vi "Deserialize Connection Info.vi"(7 "Field Delimiter (::)":string="::", 8 "error in (no error)":errorcluster, 11 "Connection Info String":string) -> (0 "error out":errorcluster, 3 "Deserialized Connection Info":T1)   [LabVIEW 2020, in "plugin_flodx_ph_probe.lvlib" / "plugin.lvlib" / "Instrument Manager.lvlib"]
doc: "Deserializes a connection info string. By default, it deserializes a string in the format \"<visa_resource>::<pump_address>\"."
uses:
  Instrument Manager.lvlib
  Connection Info.ctl
panel:
  out "homogenized string":string
  # "Debug"
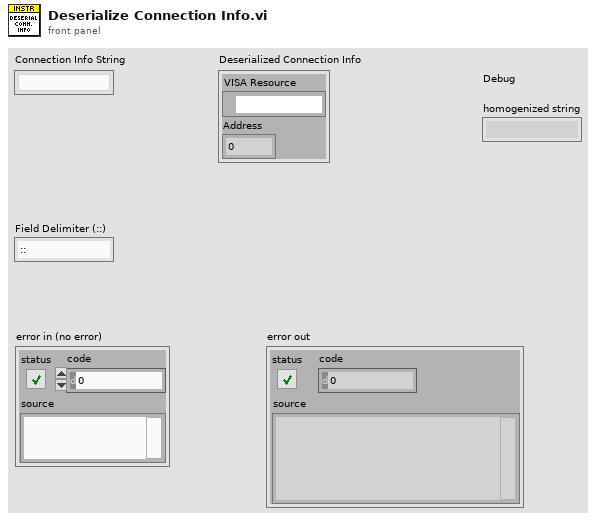
[diagram p1: front panel]
types:
  T1 = typedef "plugin_flodx_ph_probe.lvlib/plugin.lvlib/Instrument Manager.lvlib/Connection Info.ctl" = cluster{"VISA Resource":refnum<visa-resource-name>, "Address":u8}
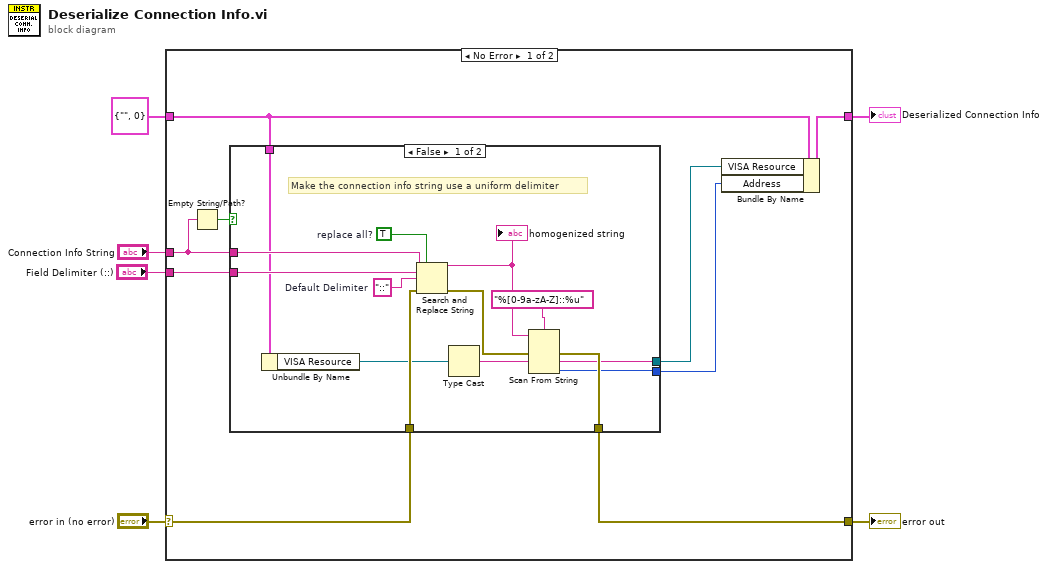
[diagram p0: block diagram]
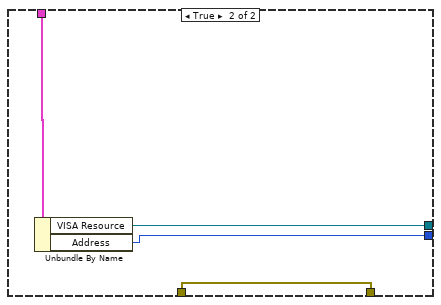
[diagram p2: hidden frame]
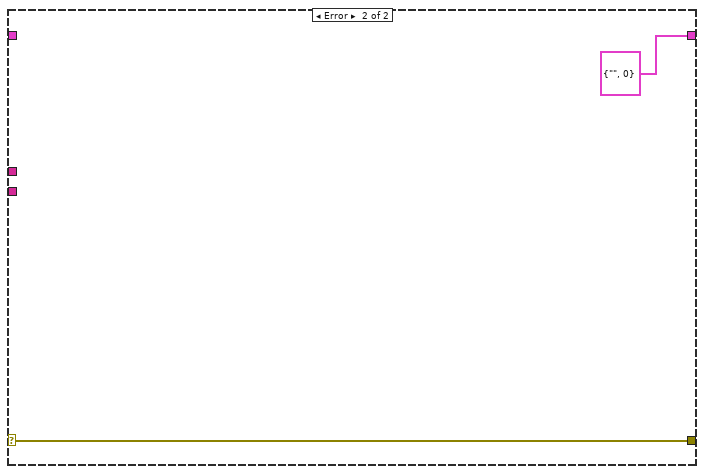
[diagram p3: hidden frame]
diagram:
  n1 = case shown="No Error" "error in (no error)" {
    selector: "error in (no error)" -> [w14 w35]
    tunnel: [w15 w35] -> w5
    tunnel: "Field Delimiter (::)" -> [w13 _]
    tunnel: [w12 T1 {"VISA Resource"="", "Address"=0} ("Deserialized Connection Info")] -> w3
    tunnel: "Connection Info String" -> [w8 _]
    tunnel: T1 {"VISA Resource"="", "Address"=0} ("Deserialized Connection Info") -> [w10 _]
    frame No Error {
      n2 = Empty String/Path?(string/path=w8) -> (empty?=w9:bool)
      n3 = case shown="False" w9 {
        tunnel: [w29 w31] -> w15
        tunnel: w14 -> [w28 w31]
        tunnel: w8 -> [w23 _]
        tunnel: w13 -> [w22 _]
        tunnel: [w19 w32] -> w11
        tunnel: w10 -> [w17 w33]
        tunnel: [w16 w30] -> w7
        frame False {
          w26 = TRUE  # replace all?
          w21 = "::"  # Default Delimiter
          # "Make the connection info string use a uniform delimiter"
          n4 = Unbundle By Name(w17) -> ("VISA Resource"=w25:refnum<visa-resource-name>)
          n5 = Search and Replace String(replace all?=w26, input string=w23, search string=w22, replace string=w21, error in=w28) -> (result string=w18:string, error out=w27:errorcluster)  [unwired: 3 in, 2 out]
          "homogenized string" <- w18
          n6 = Type Cast(x=w25) -> (*(type *) &x=w20:string)  [unwired: 1 in]
          n7 = Scan From String(format string="%[0-9a-zA-Z]::%u" ("Format String"), input string=w18, error in=w27, default 1=w20) -> (error out=w29:errorcluster, output 1=w19:string, output 2=w16:u32)  [unwired: 2 in, 2 out]
        }
        frame True {
          n8 = Unbundle By Name(w33) -> ("VISA Resource"=w32:refnum<visa-resource-name>, "Address"=w30:u8)
        }
      }
      n9 = Bundle By Name(cluster=w10, "VISA Resource"=w11, "Address"=w7) -> (w12:T1)
    }
    frame Error {
    }
  }
  "error out" <- w5
  "Deserialized Connection Info" <- w3
